vi "Write Numeric.vi"(8 "error in (no error)":errorcluster, 10 "Numeric":i32, 11 "BasicTerminalBinding in":refnum<class "BasicTerminalBinding.lvclass">) -> (0 "error out":errorcluster, 3 "BasicTerminalBinding out":refnum<class "BasicTerminalBinding.lvclass">)   [LabVIEW 2020, in "TestViewables.lvlib" / "BasicTerminalBinding.lvclass"]
uses:
  BasicTerminalBinding.lvclass
  BasicTerminalBinding.lvclass/BasicTerminalBinding.ctl
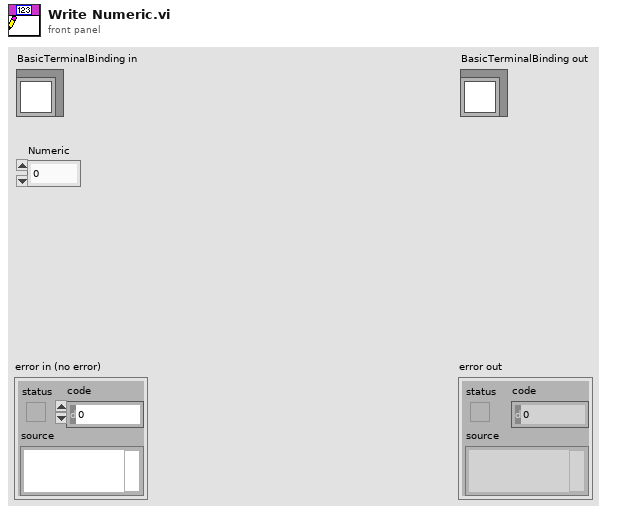
[diagram p1: front panel]
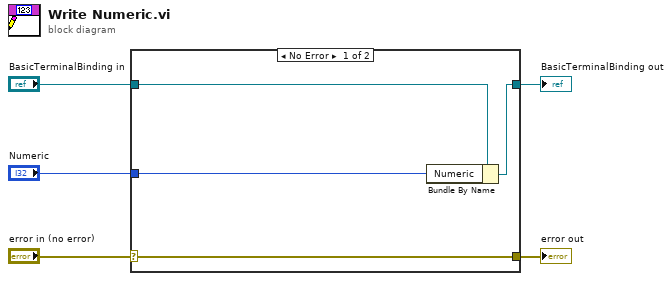
[diagram p0: block diagram]
diagram:
  n1 = case shown="No Error" "error in (no error)" {
    selector: "error in (no error)" -> [w9 w10]
    tunnel: [w9 w10] -> w4
    tunnel: [w7 w11] -> w2
    tunnel: "BasicTerminalBinding in" -> [w8 w11]
    tunnel: "Numeric" -> [w6 _]
    frame No Error {
      n2 = Bundle By Name(cluster=w8, "Numeric"=w6) -> (w7:refnum<class "BasicTerminalBinding.lvclass">)
    }
    frame Error {
    }
  }
  "error out" <- w4
  "BasicTerminalBinding out" <- w2
